vi "Game Map.vi"() -> (5 "MAP1":T1={"Game Road 1"=1, "Game Road 2"=1, "Game Road 3"=1, "Game Road 4"=1, "Game Road 5"=1, "Game Road 6"=1, "Game Road 7"=0, "Game Road 8"=1, "Game Road 9"=1, "Game Road 10"=1, "Game Road 11"=1, "Game Road 12"=2, "Game Road 13"=1, "Game Road 14"=1, "Game Road 15"=0, "Game Coin 1"=1, "Game Coin 2"=1, "Game Coin 3"=1, "Game Coin 4"=1, "Game Coin 5"=1, "Game Coin 6"=1, "Game Coin 7"=1, "Game Coin 8"=1, "Game Coin 9"=1, "Game Coin 10"=1, "Game Coin 11"=1, "Game Coin 12"=1, "Game Coin 13"=1, "Game Coin 14"=1, "Game Coin 15"=1, "Game Coin 16"=1, "Game Coin 17"=1, "Game Coin 18"=1, "Game Coin 19"=1, "Game Coin 20"=1, "Game Coin 21"=1, "Game Coin 22"=1, "Game Coin 23"=1, "Game Coin 24"=2, "Game Coin 25"=2, "Game Coin 26"=2, "Game Coin 27"=2, "Game Coin 28"=2, "Game Coin 29"=2, "Game Coin 30"=1, "Game Coin 31"=1, "Game Coin 32"=1, "Game Coin 33"=1, "Game Coin 34"=1, "Game Coin 35"=1, "Game Coin 36"=1, "Game Coin 37"=1, "Game Coin 38"=1, "Game Coin 39"=1, "Game Coin 40"=2, "Game Coin 41"=2, "Game Coin 42"=2, "Game Coin 43"=2, "Game Coin 44"=1, "Game Coin 45"=1, "Game Coin 46"=1, "Game Coin 47"=1, "Game Coin 48"=1, "Game Coin 49"=1, "Game Coin 50"=2, "Game Coin 51"=2, "Game Coin 52"=2, "Game Coin 53"=2, "Game Coin 54"=2, "Game Coin 55"=2, "Game Coin 56"=2, "Game Coin 57"=2, "Game Coin 58"=2, "Game Coin 59"=2, "Game Coin 60"=2}, 6 "MAP2":T1={"Game Road 1"=1, "Game Road 2"=1, "Game Road 3"=0, "Game Road 4"=1, "Game Road 5"=1, "Game Road 6"=1, "Game Road 7"=2, "Game Road 8"=1, "Game Road 9"=1, "Game Road 10"=1, "Game Road 11"=1, "Game Road 12"=1, "Game Road 13"=1, "Game Road 14"=1, "Game Road 15"=0, "Game Coin 1"=1, "Game Coin 2"=1, "Game Coin 3"=1, "Game Coin 4"=1, "Game Coin 5"=1, "Game Coin 6"=1, "Game Coin 7"=1, "Game Coin 8"=1, "Game Coin 9"=2, "Game Coin 10"=2, "Game Coin 11"=2, "Game Coin 12"=2, "Game Coin 13"=1, "Game Coin 14"=1, "Game Coin 15"=1, "Game Coin 16"=1, "Game Coin 17"=1, "Game Coin 18"=1, "Game Coin 19"=1, "Game Coin 20"=1, "Game Coin 21"=2, "Game Coin 22"=2, "Game Coin 23"=2, "Game Coin 24"=2, "Game Coin 25"=2, "Game Coin 26"=2, "Game Coin 27"=2, "Game Coin 28"=2, "Game Coin 29"=2, "Game Coin 30"=2, "Game Coin 31"=2, "Game Coin 32"=2, "Game Coin 33"=1, "Game Coin 34"=1, "Game Coin 35"=1, "Game Coin 36"=1, "Game Coin 37"=1, "Game Coin 38"=1, "Game Coin 39"=1, "Game Coin 40"=1, "Game Coin 41"=1, "Game Coin 42"=1, "Game Coin 43"=1, "Game Coin 44"=1, "Game Coin 45"=1, "Game Coin 46"=1, "Game Coin 47"=1, "Game Coin 48"=1, "Game Coin 49"=1, "Game Coin 50"=1, "Game Coin 51"=2, "Game Coin 52"=2, "Game Coin 53"=2, "Game Coin 54"=2, "Game Coin 55"=2, "Game Coin 56"=2, "Game Coin 57"=2, "Game Coin 58"=2, "Game Coin 59"=2, "Game Coin 60"=2}, 7 "MAP3":T1={"Game Road 1"=1, "Game Road 2"=1, "Game Road 3"=1, "Game Road 4"=1, "Game Road 5"=1, "Game Road 6"=1, "Game Road 7"=0, "Game Road 8"=1, "Game Road 9"=1, "Game Road 10"=1, "Game Road 11"=2, "Game Road 12"=1, "Game Road 13"=1, "Game Road 14"=1, "Game Road 15"=0, "Game Coin 1"=1, "Game Coin 2"=1, "Game Coin 3"=1, "Game Coin 4"=1, "Game Coin 5"=1, "Game Coin 6"=1, "Game Coin 7"=1, "Game Coin 8"=1, "Game Coin 9"=1, "Game Coin 10"=1, "Game Coin 11"=1, "Game Coin 12"=1, "Game Coin 13"=1, "Game Coin 14"=1, "Game Coin 15"=1, "Game Coin 16"=1, "Game Coin 17"=1, "Game Coin 18"=1, "Game Coin 19"=1, "Game Coin 20"=1, "Game Coin 21"=1, "Game Coin 22"=1, "Game Coin 23"=1, "Game Coin 24"=2, "Game Coin 25"=2, "Game Coin 26"=2, "Game Coin 27"=2, "Game Coin 28"=2, "Game Coin 29"=2, "Game Coin 30"=2, "Game Coin 31"=1, "Game Coin 32"=1, "Game Coin 33"=1, "Game Coin 34"=1, "Game Coin 35"=1, "Game Coin 36"=1, "Game Coin 37"=1, "Game Coin 38"=1, "Game Coin 39"=1, "Game Coin 40"=1, "Game Coin 41"=2, "Game Coin 42"=2, "Game Coin 43"=2, "Game Coin 44"=2, "Game Coin 45"=1, "Game Coin 46"=1, "Game Coin 47"=1, "Game Coin 48"=1, "Game Coin 49"=1, "Game Coin 50"=1, "Game Coin 51"=1, "Game Coin 52"=1, "Game Coin 53"=1, "Game Coin 54"=1, "Game Coin 55"=2, "Game Coin 56"=2, "Game Coin 57"=2, "Game Coin 58"=2, "Game Coin 59"=2, "Game Coin 60"=2})   [LabVIEW 2010]
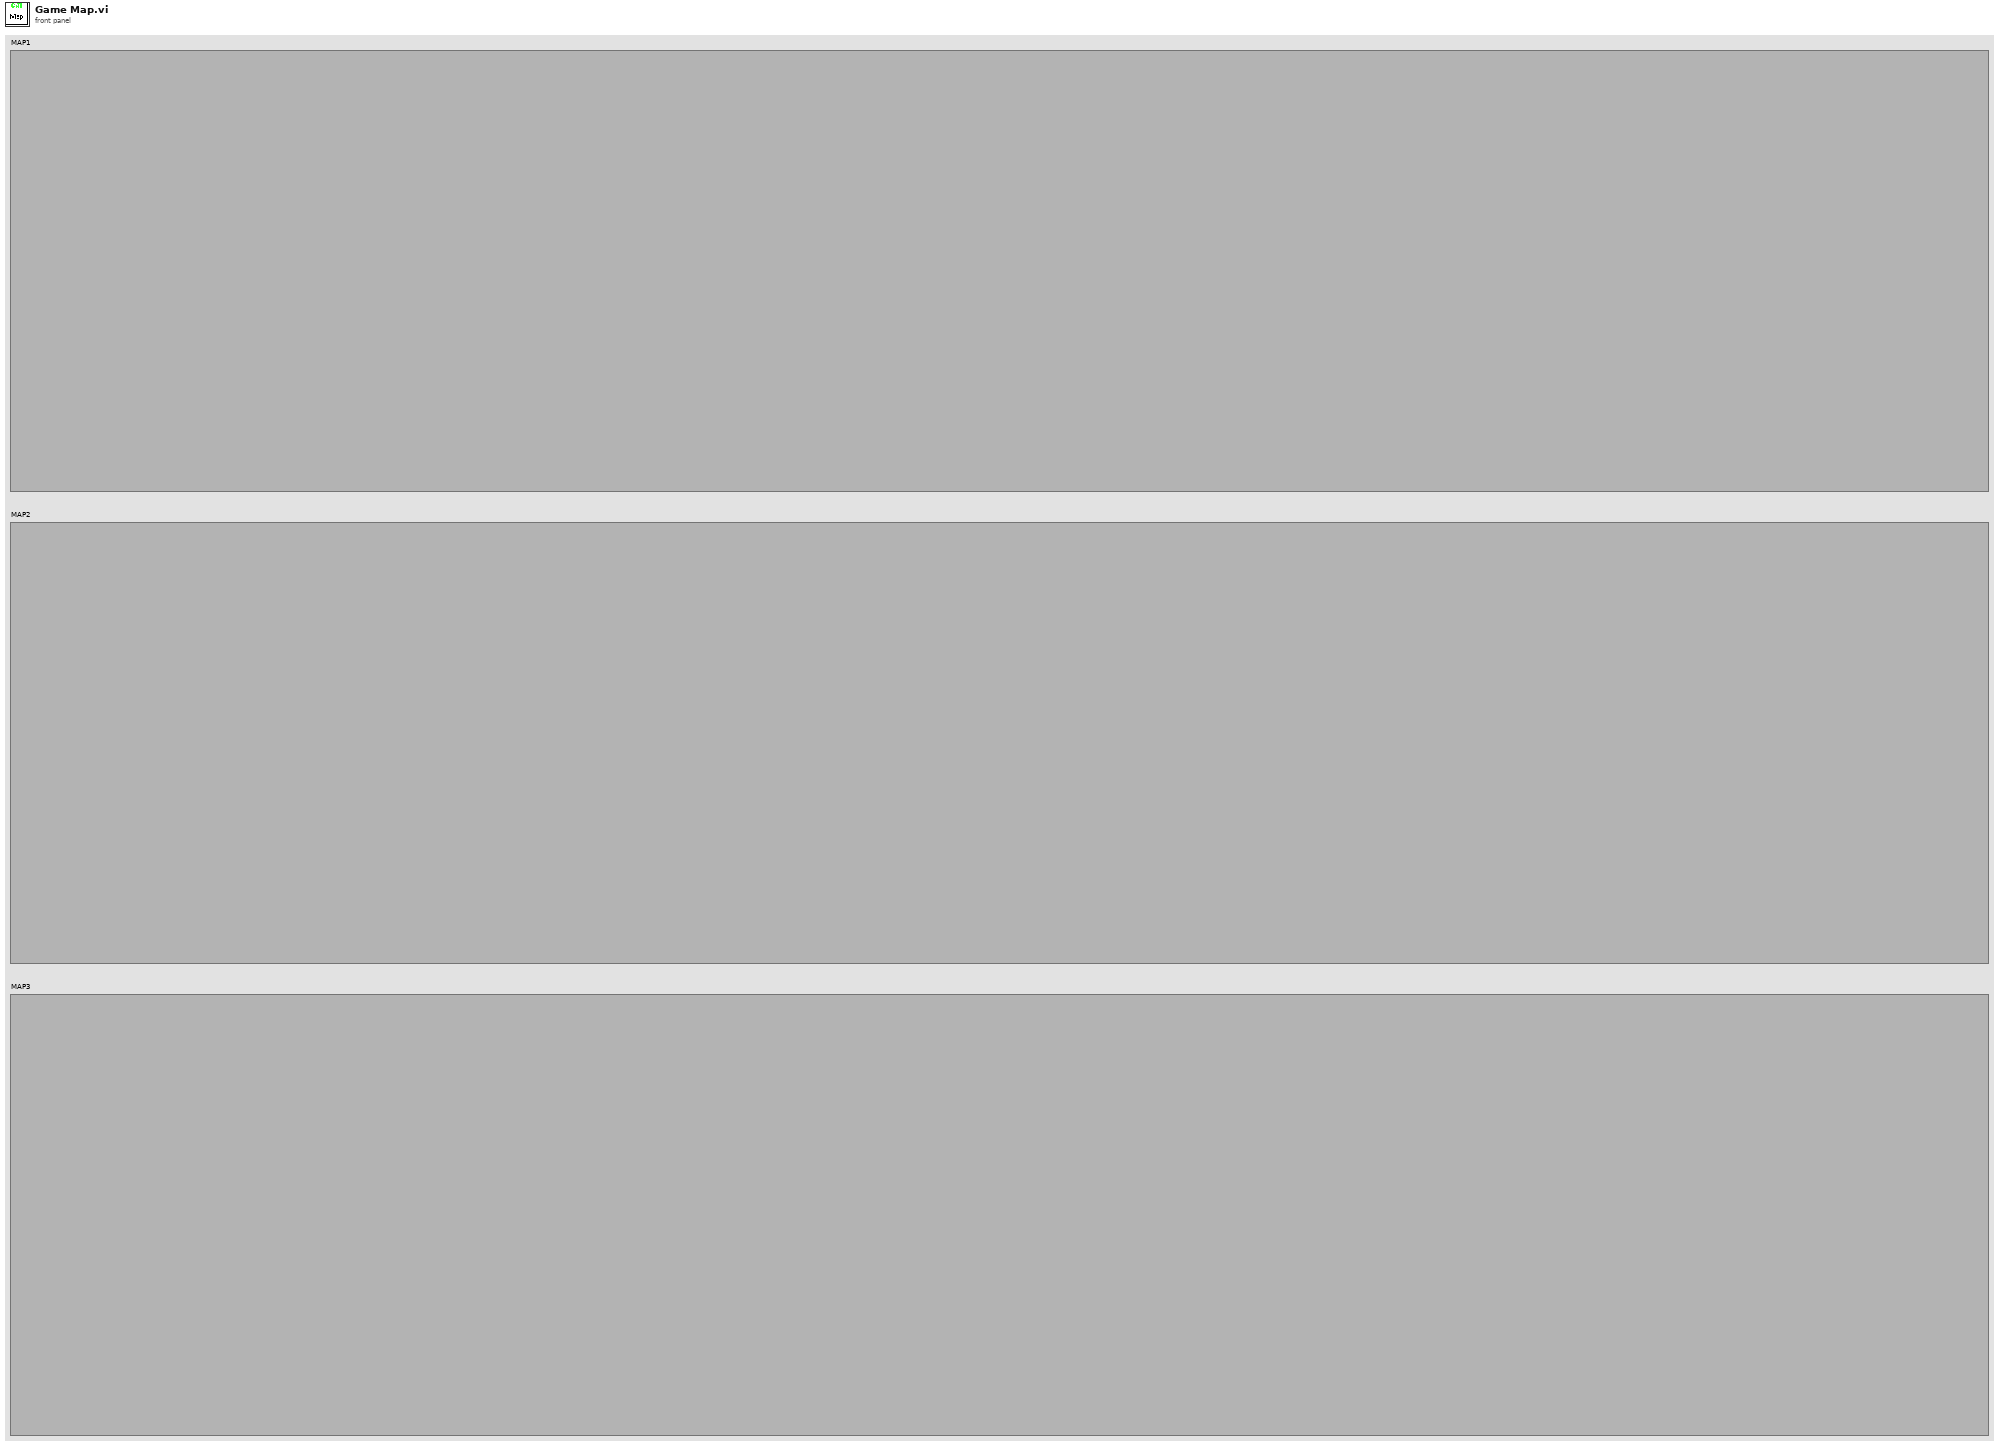
[diagram p1: front panel]
types:
  T1 = cluster{"Game Road 1":u16, "Game Road 2":u16, "Game Road 3":u16, "Game Road 4":u16, "Game Road 5":u16, "Game Road 6":u16, "Game Road 7":u16, "Game Road 8":u16, "Game Road 9":u16, "Game Road 10":u16, "Game Road 11":u16, "Game Road 12":u16, "Game Road 13":u16, "Game Road 14":u16, "Game Road 15":u16, "Game Coin 1":u16, "Game Coin 2":u16, "Game Coin 3":u16, "Game Coin 4":u16, "Game Coin 5":u16, "Game Coin 6":u16, "Game Coin 7":u16, "Game Coin 8":u16, "Game Coin 9":u16, "Game Coin 10":u16, "Game Coin 11":u16, "Game Coin 12":u16, "Game Coin 13":u16, "Game Coin 14":u16, "Game Coin 15":u16, "Game Coin 16":u16, "Game Coin 17":u16, "Game Coin 18":u16, "Game Coin 19":u16, "Game Coin 20":u16, "Game Coin 21":u16, "Game Coin 22":u16, "Game Coin 23":u16, "Game Coin 24":u16, "Game Coin 25":u16, "Game Coin 26":u16, "Game Coin 27":u16, "Game Coin 28":u16, "Game Coin 29":u16, "Game Coin 30":u16, "Game Coin 31":u16, "Game Coin 32":u16, "Game Coin 33":u16, "Game Coin 34":u16, "Game Coin 35":u16, "Game Coin 36":u16, "Game Coin 37":u16, "Game Coin 38":u16, "Game Coin 39":u16, "Game Coin 40":u16, "Game Coin 41":u16, "Game Coin 42":u16, "Game Coin 43":u16, "Game Coin 44":u16, "Game Coin 45":u16, "Game Coin 46":u16, "Game Coin 47":u16, "Game Coin 48":u16, "Game Coin 49":u16, "Game Coin 50":u16, "Game Coin 51":u16, "Game Coin 52":u16, "Game Coin 53":u16, "Game Coin 54":u16, "Game Coin 55":u16, "Game Coin 56":u16, "Game Coin 57":u16, "Game Coin 58":u16, "Game Coin 59":u16, "Game Coin 60":u16}
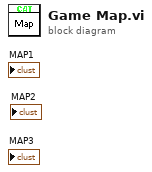
[diagram p0: block diagram]
diagram:
